vi "asyncViStopsFromAbortedOutput.vi"(10 "subchannel (0)":i32, 11 "channel":T1) -> (3 "other channel":T1)   [LabVIEW 2020, in "Tests Event MessengerM.lvclass"]
uses:
  Tests Event MessengerM.lvclass
  <extravilib>/ChannelInstances/Event MessengerM-i32/))Channel.ctl
  <extravilib>/ChannelInstances/Event MessengerM-i32/))Channel.vi
  <extravilib>/ChannelInstances/Event MessengerM-i32.lvlib
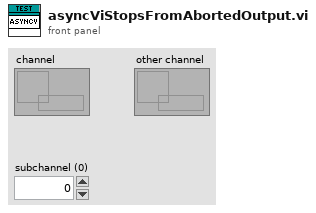
[diagram p1: front panel]
types:
  T1 = typedef "Event MessengerM-i32.lvlib/))Channel.ctl" = refnum<queue>
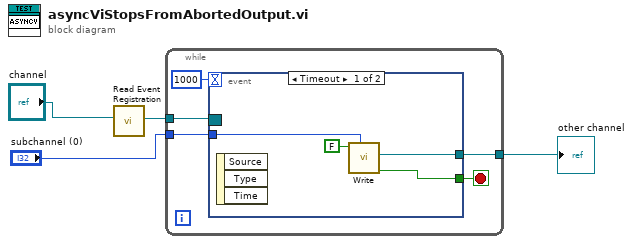
[diagram p0: block diagram]
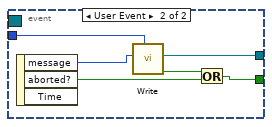
[diagram p2: hidden frame]
diagram:
  n1 = call <extravilib>:"Read Event Registration.vi"("channel"="channel") -> ("event registration refnum"=w2:refnum<event-registration>)  [unwired: 10 in]
  n2 = while {
    tunnel: w2 -> [w9]
    tunnel: "subchannel (0)" -> [w7]
    tunnel: [w5] -> w1
    stop <- w8 stop-if-true
    n3 = event shown="[0] Timeout" {
      selector: w9 -> [_ _]
      dyn-events: _ -> [_ _]
      timeout: 1000 -> [_ _]
      tunnel: [w12 w18] -> w8
      tunnel: w7 -> [w13 w17]
      tunnel: [w11 w16] -> w5
      event Timeout {
        n4 = event-data() -> ()  [unwired: 1 in, 3 out]
        n5 = call <extravilib>:"Write.vi"("subchannel (0)"=w13, "element valid? (T)"=FALSE) -> ("done?"=w12:bool, "channel"=w11:T1)  [unwired: 8 in]
      }
      event User Event {
        n6 = event-data() -> ("message"=w14:i32, "aborted?"=w19:bool)  [unwired: 1 in, 1 out]
        n7 = call <extravilib>:"Write.vi"("subchannel (0)"=w17, "element"=w14) -> ("done?"=w15:bool, "channel"=w16:T1)  [unwired: 8 in]
        n8 = Or(x=w15, y=w19) -> (x .or. y?=w18:bool)
      }
    }
  }
  "other channel" <- w1
